vi "通用Get.vi"(8 "error in (no error)":errorcluster caption="错误输入（无错误）", 11 "MainPage 输入":refnum<class "MainPage.lvclass">) -> (0 "error out":errorcluster caption="错误输出", 1 "非法引用句柄？":bool, 2 "通用配置":T1={"ModBusRTU反馈"=enum."无反馈", "侦听周期"=0, "跳转反馈"=FALSE, "报文记录数量"=0, "客服端新增模式"=enum."单端模式"}, 3 "MainPage 输出":refnum<class "MainPage.lvclass">, 4 "通用引用":refnum<data-value>)   [LabVIEW 2019, in "MainPage.lvlib" / "MainPage.lvclass"]
uses:
  MainPage.lvclass
  MainPage.lvclass/MainPage.ctl
panel:
  # "实际+10ms间隔时间"
  # "达到上限会顶替旧记录"
  # "实际+10ms间隔时间"
  # "达到上限会顶替旧记录"
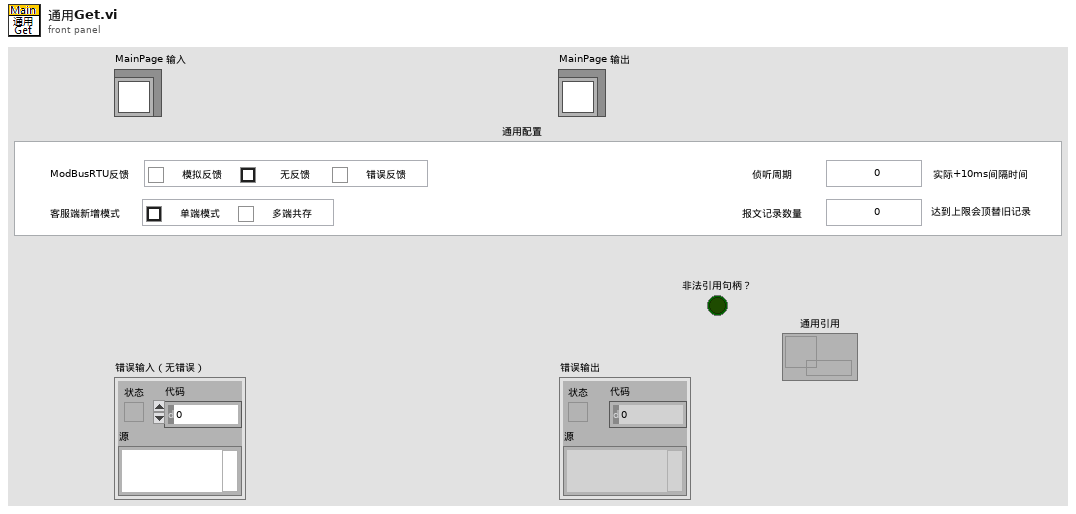
[diagram p1: front panel]
types:
  T1 = typedef "MainPage.lvlib/MainPage.lvclass/通用配置选项.ctl" = cluster{"ModBusRTU反馈":enum32{"模拟反馈", "无反馈", "错误反馈"}, "侦听周期":u32, "跳转反馈":bool, "报文记录数量":u16, "客服端新增模式":enum32{"单端模式", "多端共存"}}
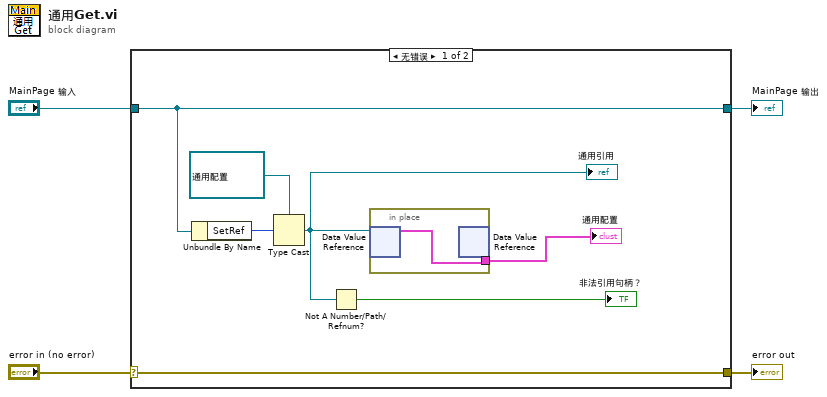
[diagram p0: block diagram]
diagram:
  n1 = case shown="无错误" "error in (no error)" {
    selector: "error in (no error)" -> [w11 w14]
    tunnel: [w11 w14] -> w3
    tunnel: [w10 w13] -> w1
    tunnel: "MainPage 输入" -> [w10 w13]
    frame No Error {
      n2 = Unbundle By Name(w10) -> ("SetRef"=w8:u32)
      n3 = Type Cast(type=refnum<data-value> refnum ("通用引用"), x=w8) -> (*(type *) &x=w6:refnum<data-value>)
      "通用引用" <- w6
      n4 = Not A Number/Path/Refnum?(number/path/refnum=w6) -> (NaN/Path/Refnum?=→"非法引用句柄？":bool)
      n5 = in-place {
        in-place-border: [w12] -> w5
        n6 = in-place-dvr #1(w6) -> (w12:T1)  [unwired: 1 out]
        n7 = in-place-dvr #1() -> ()  [unwired: 1 in, 2 out]
      }
      "通用配置" <- w5
    }
    frame Error {
    }
  }
  "error out" <- w3
  "MainPage 输出" <- w1
